vi "AdvServoEventExe.vi"(8 "error in (no error)":errorcluster, 10 "Event Registration Refnum In":refnum<event-registration>, 11 "Device In":i32) -> (0 "error out":errorcluster, 1 "index":i32, 2 "Event Registration Refnum Out":refnum<event-registration>, 3 "Device Out":i32, 4 "Value":dbl, 5 "Event?":bool)   [LabVIEW 2012]
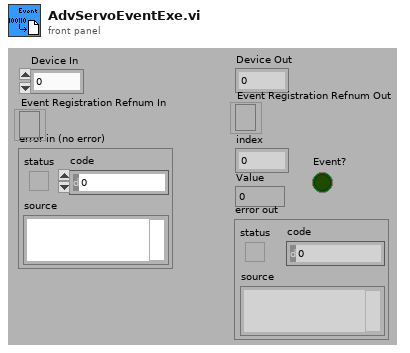
[diagram p1: front panel]
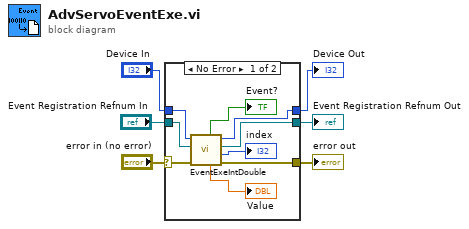
[diagram p0: block diagram]
diagram:
  n1 = case shown="No Error" "error in (no error)" {
    selector: "error in (no error)" -> [w15 w18]
    tunnel: [w10 w18] -> w5
    tunnel: "Device In" -> [w14 w17]
    tunnel: [w13 w17] -> w3
    tunnel: [w11 w16] -> w2
    tunnel: "Event Registration Refnum In" -> [w12 w16]
    frame No Error {
      n2 = call "EventExeIntDouble.vi"("error in (no error)"=w15, "Event Registration Refnum In"=w12, "Device In"=w14) -> ("error out"=w10:errorcluster, "index"=→"index":i32, "Event Registration Refnum Out"=w11:refnum<event-registration>, "Device Out"=w13:i32, "acceleration"=→"Value":dbl, "Event?"=→"Event?":bool)  [unwired: 3 in]
    }
    frame Error {
    }
  }
  "Device Out" <- w3
  "error out" <- w5
  "Event Registration Refnum Out" <- w2
